vi "Eurotherm - Simple Front Panel Control.vi"(0 "Setup":T1={"Communication"={"Com Port"=1, "Address"=1, "Baud Rate"=9600}, "Name"="", "Enable"=FALSE, "Max Set Point"=0.0, "Min Set Point"=0.0, "Units"="", "Graph Data"=0, "Sensor type"=enum."RhFe", "Calibration File Path"=path "", "Conversion Type"=enum."Linear"} {"Min Set Point" format="%.3f"; "Max Set Point" format="%.3f"; "Communication"."Baud Rate" items=["300"=300, "600"=600, "1200"=1200, "2400"=2400, "4800"=4800, "9600 (default)"=9600, "19200"=19200, "38400"=38400, "57600"=57600, "76800"=76800, "115200"=115200, "230400"=230400]; "Communication"."Com Port" min=1 max=255; "Communication"."Address" min=1 max=99}, 1 "Temperature":refnum<vi>, 2 "Setpoint":refnum<vi>, 11 "error in (no error)":errorcluster, 12 "Set":refnum<vi>, 13 "Required Setpoint":refnum<vi>) -> (15 "error out":errorcluster)   [LabVIEW 2011]
uses:
  Eurotherm - Controls/Eurotherm - Setup.ctl
  Eurotherm - Controls/Eurotherm - Communication.ctl
  Common/Utilities/Controls - Com Ports/Com Port - Numeric.ctl
  Eurotherm - Controls/Eurotherm - Address.ctl
  Common/Utilities/Controls - Com Ports/Com Port - Baud Rate.ctl
  Common/Utilities - System/Sensors/Sensors - Controls/Sensors - Temperature Sensor Type.ctl
  Common/Utilities - System/Sensors/Sensors - Controls/Sensors - Conversion Type.ctl
  Common/Utilities/Event Log/Event Log - Priority.ctl
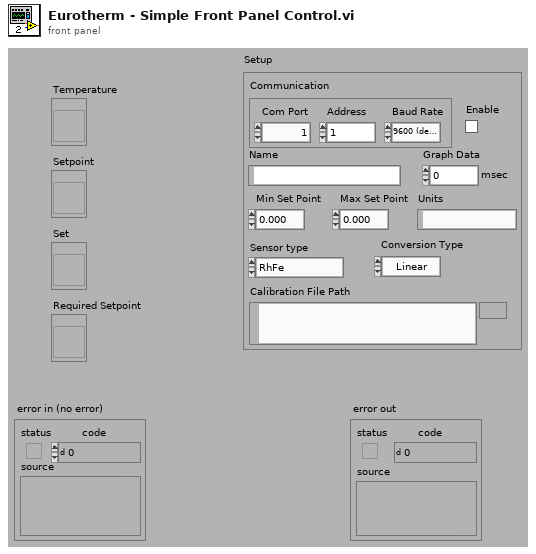
[diagram p1: front panel]
types:
  T1 = typedef "Eurotherm - Setup.ctl" = cluster{"Communication":T2, "Name":string, "Enable":bool, "Max Set Point":dbl, "Min Set Point":dbl, "Units":string, "Graph Data":u32, "Sensor type":T6, "Calibration File Path":path, "Conversion Type":T7}
  T2 = typedef "Eurotherm - Communication.ctl" = cluster{"Com Port":T3, "Address":T4, "Baud Rate":T5}
  T3 = typedef "Com Port - Numeric.ctl" = i32
  T4 = typedef "Eurotherm - Address.ctl" = u8
  T5 = typedef "Com Port - Baud Rate.ctl" = u32
  T6 = typedef "Sensors - Temperature Sensor Type.ctl" = enum16{"RhFe", "Pt", "K type thermocouple", "W5 type thermocouple", "No Conversion"}
  T7 = typedef "Sensors - Conversion Type.ctl" = enum16{"Linear", "Spline"}
  T8 = typedef "Event Log - Priority.ctl" = enum16{"None", "Log", "SECI and Log"}
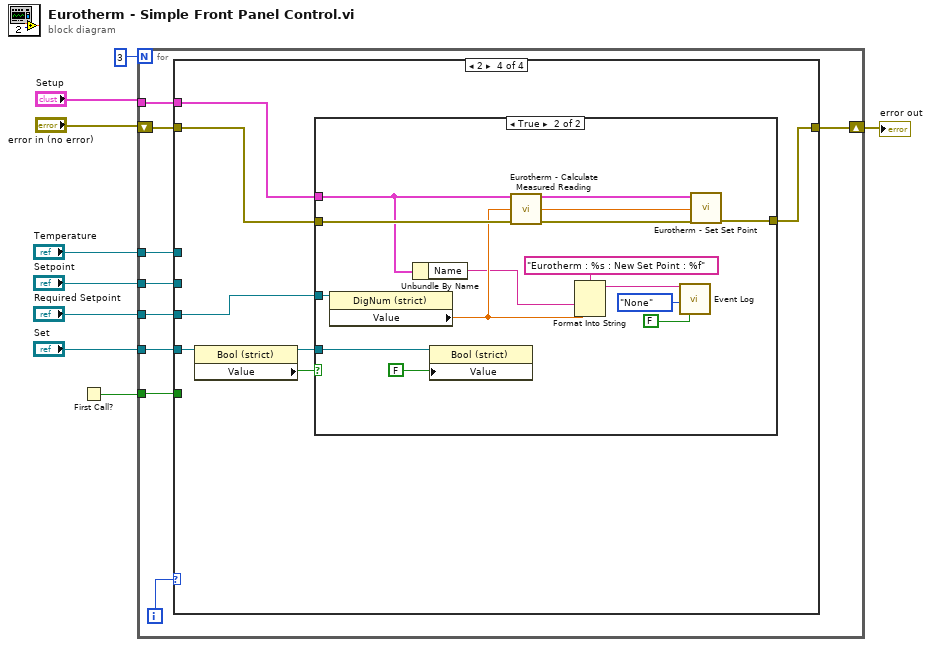
[diagram p0: block diagram]
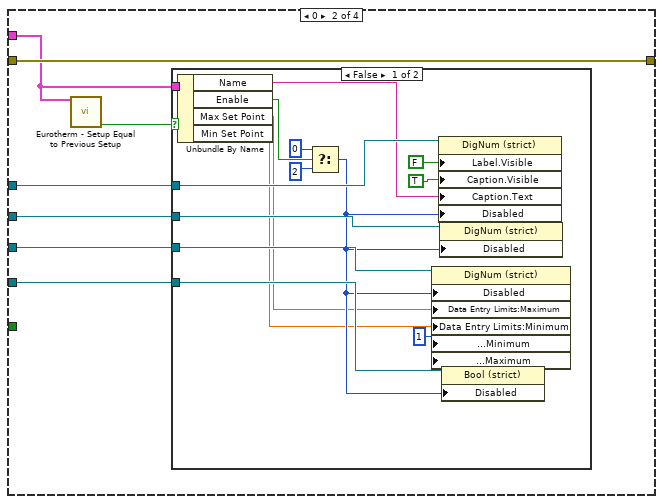
[diagram p3: hidden frame]
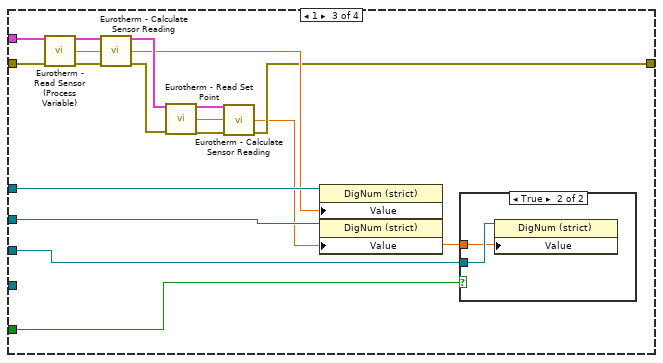
[diagram p5: hidden frame]
diagram:
  n1 = First Call?() -> (First Call?: T/F=w1:bool)
  n2 = for {
    N: 3 -> [_]
    shift-right: [w13] -> w5
    shift-left: "error in (no error)" -> [w17]
    tunnel: "Setup" -> [w18]
    tunnel: "Temperature" -> [w15]
    tunnel: "Setpoint" -> [w14]
    tunnel: "Required Setpoint" -> [w12]
    tunnel: "Set" -> [w11]
    tunnel: w1 -> [w10]
    i -> [w16]
    n3 = case shown="2" w16 {
      tunnel: w18 -> [_ w21 w58 w62]
      tunnel: w17 -> [w19 w26 w57 w63]
      tunnel: w15 -> [_ w25 w56 _]
      tunnel: w14 -> [_ w24 w55 _]
      tunnel: [w19 w26 w45 w61] -> w13
      tunnel: w12 -> [_ w23 w44 w64]
      tunnel: w11 -> [_ w22 _ w67]
      tunnel: w10 -> [_ _ w42 _]
      frame Default {
      }
      frame 0 {
        n4 = call "Eurotherm - Setup Equal to Previous Setup.vi"("Value In"=w21) -> ("Equal to previous value"=w20:bool)  [unwired: 13 in, 1 out]
        n5 = case shown="False" w20 {
          tunnel: w21 -> [w41 _]
          tunnel: w25 -> [w40 _]
          tunnel: w24 -> [w39 _]
          tunnel: w23 -> [w38 _]
          tunnel: w22 -> [w37 _]
          frame False {
            w29 = u8 1 ("Out Of Range Action:Minimum")
            n6 = Unbundle By Name(w41) -> ("Name"=w32:string, "Enable"=w33:bool, "Max Set Point"=w28:dbl, "Min Set Point"=w27:dbl)
            n7 = Select(t=u8 0 ("Disabled"), s=w33, f=u8 2 ("Disabled")) -> (s? t:f=w34:u8)
            n8 = property class="DigNum (strict)"(reference=w38, "Disabled"=w34, "Data Entry Limits:Maximum"=w28, "Data Entry Limits:Minimum"=w27, "Response to Value Outside Limits:Minimum"=w29, "Response to Value Outside Limits:Maximum"=w29) -> ()  [unwired: 1 in, 2 out]
            n9 = property class="DigNum (strict)"(reference=w40, "Label.Visible"=FALSE, "Caption.Visible"=TRUE, "Caption.Text"=w32, "Disabled"=w34) -> ()  [unwired: 1 in, 2 out]
            n10 = property class="DigNum (strict)"(reference=w39, "Disabled"=w34) -> ()  [unwired: 1 in, 2 out]
            n11 = property class="Bool (strict)"(reference=w37, "Disabled"=w34) -> ()  [unwired: 1 in, 2 out]
          }
          frame True {
          }
        }
      }
      frame 1 {
        n12 = call "Eurotherm - Read Sensor (Process Variable).vi"("Eurotherm Setup In"=w58, "error in (no error)"=w57) -> ("Eurotherm Setup Out"=w54:T1, "Reading"=w53:dbl, "error out"=w52:errorcluster)  [unwired: 11 in]
        n13 = call "Eurotherm - Calculate Sensor Reading.vi"("Eurotherm Setup In"=w54, "Measured Value"=w53, "error in (no error)"=w52) -> ("Eurotherm Setup Out"=w51:T1, "Converted Value"=w50:dbl, "error out"=w49:errorcluster)  [unwired: 10 in]
        n14 = call "Eurotherm - Read Set Point.vi"("Eurotherm Setup In"=w51, "error in (no error)"=w49) -> ("Eurotherm Setup Out"=w48:T1, "Set Point"=w47:dbl, "error out"=w46:errorcluster)  [unwired: 11 in]
        n15 = call "Eurotherm - Calculate Sensor Reading.vi"("Eurotherm Setup In"=w48, "Measured Value"=w47, "error in (no error)"=w46) -> ("Converted Value"=w43:dbl, "error out"=w45:errorcluster)  [unwired: 10 in, 1 out]
        n16 = property class="DigNum (strict)"(reference=w56, "Value"=w50) -> ()  [unwired: 1 in, 2 out]
        n17 = property class="DigNum (strict)"(reference=w55, "Value"=w43) -> ()  [unwired: 1 in, 2 out]
        n18 = case shown="True" w42 {
          tunnel: w44 -> [_ w60]
          tunnel: w43 -> [_ w59]
          frame False {
          }
          frame True {
            n19 = property class="DigNum (strict)"(reference=w60, "Value"=w59) -> ()  [unwired: 1 in, 2 out]
          }
        }
      }
      frame 2 {
        n20 = property class="Bool (strict)"(reference=w67) -> (reference out=w65:refnum<vi>, "Value"=w66:bool)  [unwired: 1 in, 1 out]
        n21 = case shown="True" w66 {
          tunnel: w65 -> [_ w80]
          tunnel: w64 -> [_ w78]
          tunnel: w63 -> [w68 w77]
          tunnel: w62 -> [_ w75]
          tunnel: [w68 w76] -> w61
          frame False {
          }
          frame True {
            n22 = property class="DigNum (strict)"(reference=w78) -> ("Value"=w73:dbl)  [unwired: 1 in, 2 out]
            n23 = Unbundle By Name(w75) -> ("Name"=w72:string)
            n24 = property class="Bool (strict)"(reference=w80, "Value"=FALSE) -> ()  [unwired: 1 in, 2 out]
            n25 = call "Eurotherm - Calculate Measured Reading.vi"("Eurotherm Setup In"=w75, "Measured Value"=w73, "error in (no error)"=w77) -> ("Eurotherm Setup Out"=w83:T1, "Converted Value"=w82:dbl, "error out"=w81:errorcluster)  [unwired: 10 in]
            n26 = Format Into String(format string="Eurotherm : %s : New Set Point : %f", w72, w73) -> (resulting string=w71:string)  [unwired: 2 in, 1 out]
            n27 = call "Event Log.vi"("Event log message"=w71, "Priority"=Event_Log_-_Priority."None", "Disconnecting"=FALSE) -> ()  [unwired: 12 in, 1 out]
            n28 = call "Eurotherm - Set Set Point.vi"("Eurotherm Setup In"=w83, "Set Point"=w82, "error in (no error)"=w81) -> ("error out"=w76:errorcluster)  [unwired: 11 in, 1 out]
          }
        }
      }
    }
  }
  "error out" <- w5
